vi "RenderDiff.vi"(8 "error in (no error)":errorcluster, 11 "DiffVI in":refnum<class "DiffVI.lvclass">) -> (0 "error out":errorcluster, 3 "DiffVI out":refnum<class "DiffVI.lvclass">)   [LabVIEW 2015, in "DiffVI.lvclass"]
uses:
  DiffVI.lvclass
  DiffVI.lvclass/DiffVI.ctl
  <vilib>/lvrevbrd/ScreenshotVI.lvlib
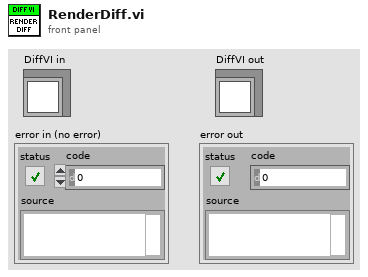
[diagram p1: front panel]
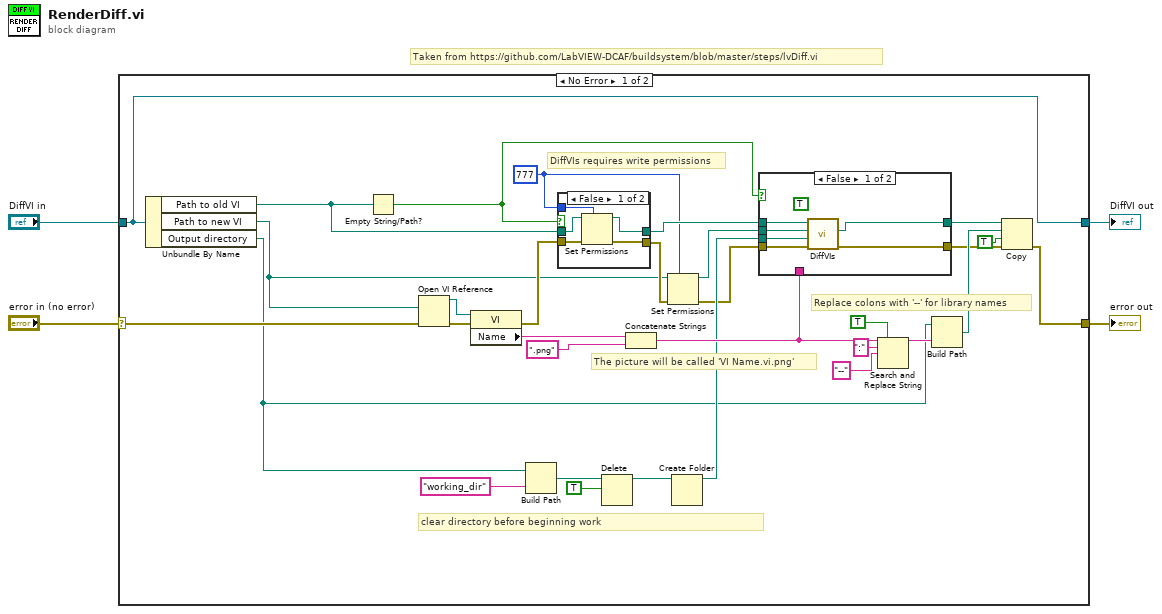
[diagram p0: block diagram]
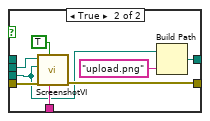
[diagram p3: hidden frame]
diagram:
  # "Taken from https://github.com/LabVIEW-DCAF/buildsystem/blob/master/steps/lvDiff.vi"
  n1 = case shown="No Error" "error in (no error)" {
    selector: "error in (no error)" -> [w35 w58]
    tunnel: [w19 w58] -> w3
    tunnel: "DiffVI in" -> [w9 w57]
    tunnel: [w9 w57] -> w1
    frame No Error {
      w20 = i16 777 ("permissions")
      # "Replace colons with '--' for library names"
      # "clear directory before beginning work"
      # "DiffVIs requires write permissions"
      # "The picture will be called 'VI Name.vi.png'"
      n2 = Unbundle By Name(w9) -> ("Path to old VI"=w5:path, "Path to new VI"=w7:path, "Output directory"=w8:path)
      n3 = Empty String/Path?(string/path=w5) -> (empty?=w6:bool)
      n4 = Open VI Reference(vi path=w7, error in (no error)=w35) -> (vi reference=w22:refnum<vi>, error out=w23:errorcluster)  [unwired: 4 in]
      n5 = property class="VI"(reference=w22, error in=w23) -> (error out=w24:errorcluster, "Name"=w25:string)  [unwired: 1 out]
      n6 = Build Path(base path=w8, name or relative path="working_dir") -> (appended path=w26:path)
      n7 = case shown="False" w6 {
        tunnel: w5 -> [w40 w41]
        tunnel: [w39 w42] -> w18
        tunnel: w20 -> [w38 _]
        tunnel: w24 -> [w37 w42]
        tunnel: [w36 w41] -> w33
        frame False {
          n8 = Set Permissions(7:w38, 8:w37, 11:w40) -> (0:w39:errorcluster, 3:w36:path)  [unwired: 2 in]
        }
        frame True {
        }
      }
      n9 = Delete(path (use dialog)=w26, entire hierarchy (F)=TRUE) -> (deleted path=w27:path)  [unwired: 3 in, 2 out]
      n10 = Concatenate Strings(w25, ".png" ("string")) -> (w32:string)
      n11 = Set Permissions(7:w20, 8:w18, 11:w7) -> (0:w10:errorcluster, 3:w11:path)  [unwired: 2 in]
      n12 = Create Folder(path (use dialog)=w27) -> (created path=w13:path)  [unwired: 2 in, 2 out]
      n13 = case shown="False" w6 {
        tunnel: w10 -> [w48 w53]
        tunnel: w11 -> [w47 w54]
        tunnel: [w46 w51] -> w12
        tunnel: w13 -> [w45 w49]
        tunnel: [w44 w55] -> w14
        tunnel: w32 -> [_ w52]
        tunnel: w33 -> [w43 _]
        frame False {
          (unwired) TRUE ("Take ScrShots All In")
          n14 = call "DiffVIs.vi"("error in"=w48, "Picture Save Location"=w45, "VI Path 2"=w47, "VI Path 1"=w43) -> ("error out"=w44:errorcluster, "diff file"=w46:path)  [unwired: 6 in]
        }
        frame True {
          n15 = call <vilib>:"ScreenshotVI.vi"("Title Prefix In"=w52, "Take Scrshots All In"=TRUE, "error in"=w53, "Picture Save Location"=w49, "VI Path"=w54) -> ("error out"=w55:errorcluster)  [unwired: 3 in, 3 out]
          n16 = Build Path(base path=w49, name or relative path="upload.png") -> (appended path=w51:path)
        }
      }
      n17 = Search and Replace String(replace all?=TRUE ("replace all? (F)"), input string=w32, search string=":", replace string="--" ("replace string (\"\")")) -> (result string=w29:string)  [unwired: 4 in, 3 out]
      n18 = Build Path(base path=w8, name or relative path=w29) -> (appended path=w17:path)
      n19 = Copy(8:w14, 9:TRUE ("overwrite (F)"), 10:w17, 11:w12) -> (0:w19:errorcluster)  [unwired: 1 in, 2 out]
    }
    frame Error {
    }
  }
  "error out" <- w3
  "DiffVI out" <- w1
